vi "multiplexer.vi"() -> ()   [LabVIEW 2014]
uses:
  <vilib>/GPower/Numeric/GPNumeric.lvlib
panel:
  in  "LogFile":path
  in  "Logging Enabled?":bool
  # "\"mplexer data in\" - queue to receive data from sensors\n\"mplexer msg in\" - queue to send messages to multiplexer\n\"mplexer clock\" - notifier that will sound off every 25 ms, with an incrementing counter as a value; use it if you like.  Also, it will be canceled 10 ms after it sounds.\n\n\n\"mplexer msg out\" - none of your business!  (holds our subscribers - internal queue)"
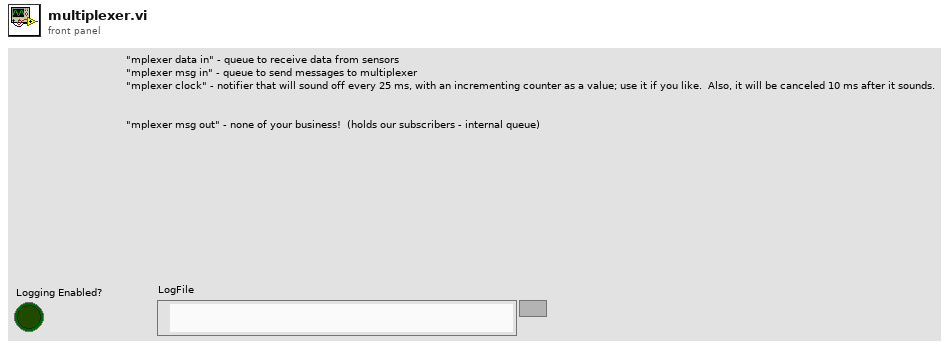
[diagram p1: front panel]
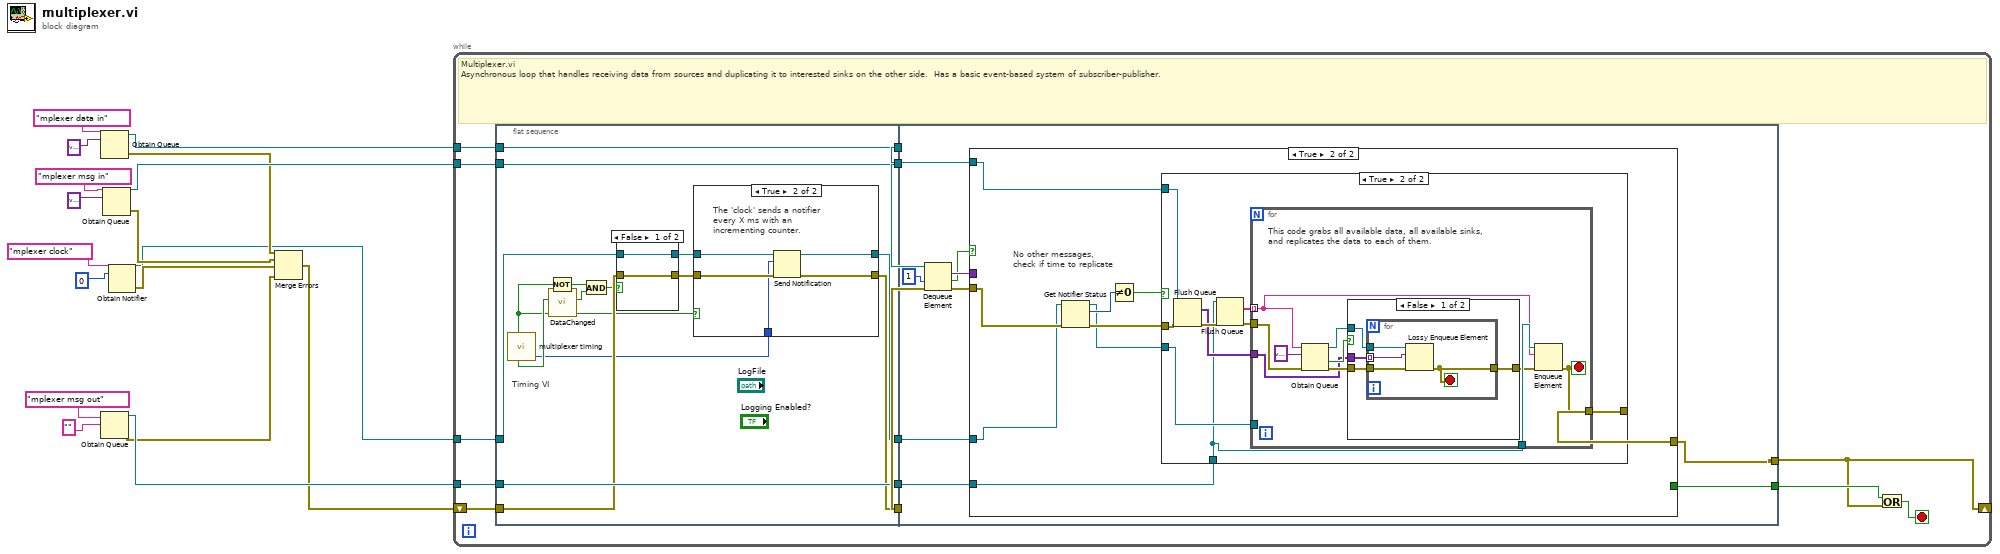
[diagram p0: block diagram]
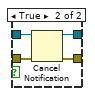
[diagram p2: hidden frame]
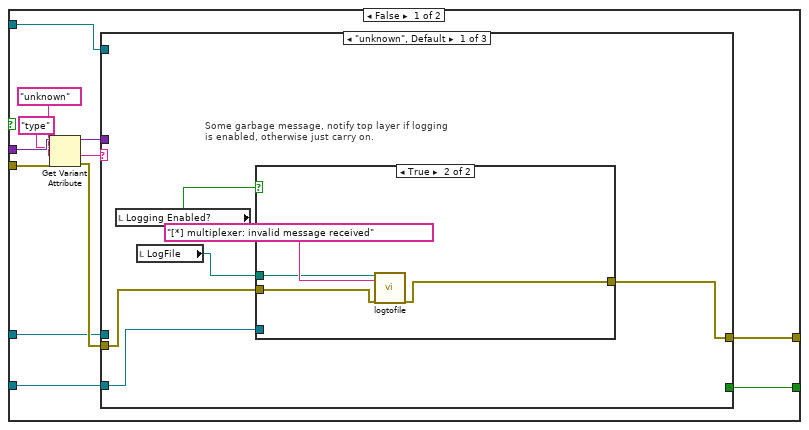
[diagram p4: hidden frame]
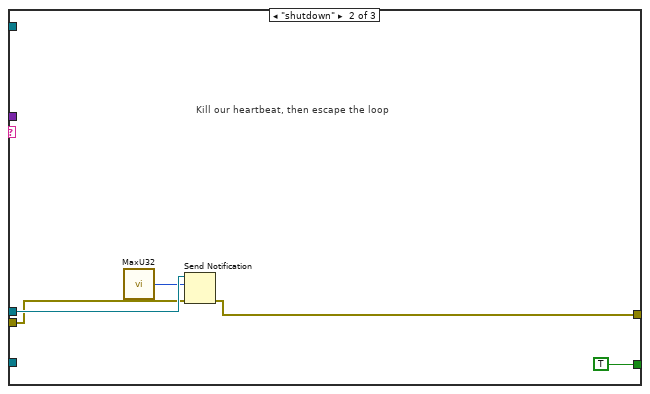
[diagram p6: hidden frame]
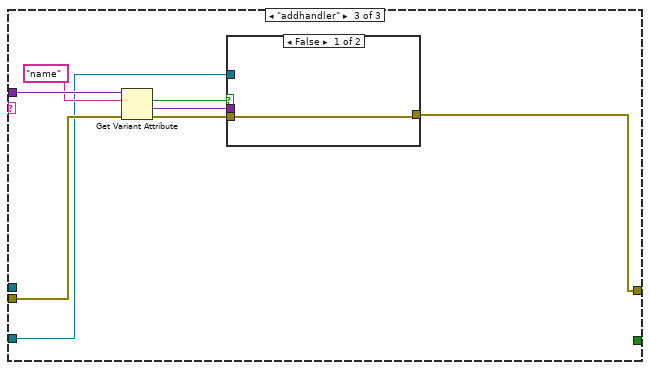
[diagram p7: hidden frame]
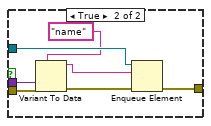
[diagram p8: hidden frame]
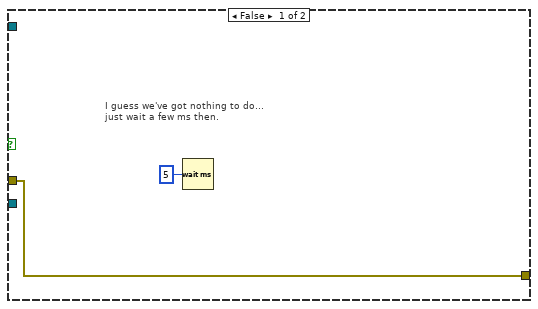
[diagram p9: hidden frame]
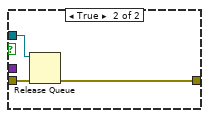
[diagram p10: hidden frame]
diagram:
  n1 = Obtain Queue(name (unnamed)="mplexer data in", element data type=variant) -> (queue out=w16:refnum<queue>, error out=w7:errorcluster)  [unwired: 3 in, 1 out]
  n2 = Obtain Queue(name (unnamed)="mplexer msg out", element data type="") -> (queue out=w13:refnum<queue>, error out=w1:errorcluster)  [unwired: 3 in, 1 out]
  n3 = Obtain Queue(name (unnamed)="mplexer msg in", element data type=variant) -> (queue out=w14:refnum<queue>, error out=w6:errorcluster)  [unwired: 3 in, 1 out]
  n4 = Obtain Notifier(name (unnamed)="mplexer clock", notification data type=u32 0) -> (notifier out=w3:refnum<notifier>, error out=w5:errorcluster)  [unwired: 2 in, 1 out]
  n5 = Merge Errors(w7, w6, w5, w1) -> (w4:errorcluster)
  n6 = while {
    tunnel: w16 -> [w20]
    shift-right: [w18] -> _
    shift-left: w4 -> [w28]
    tunnel: w14 -> [w25]
    tunnel: w13 -> [w26]
    tunnel: w3 -> [w23]
    stop <- w30 stop-if-true
    # "Multiplexer.vi\nAsynchronous loop that handles receiving data from sources and duplicating it to interested sinks on the other side.  Has a basic event-based system of subscriber-publisher."
    n7 = flat-sequence {
      tunnel: w28 -> [w40]
      tunnel: [w43] -> w29
      tunnel: [w44] -> w27
      tunnel: w26 -> [w44]
      tunnel: w25 -> [w45]
      tunnel: [w45] -> w24
      tunnel: w23 -> [w41]
      tunnel: [w32] -> w22
      tunnel: [w42] -> w21
      tunnel: w20 -> [w42]
      tunnel: w29 -> [w68]
      tunnel: w27 -> [w66]
      tunnel: w24 -> [w64]
      tunnel: [w62] -> w18
      tunnel: w22 -> [w61]
      tunnel: w21 -> [w60]
      tunnel: [w59] -> w19
      frame #0 {
        # "Timing VI"
        n8 = call "multiplexer timing.vi"() -> ("Clock Tick"=w36:bool, "Latch"=w37:bool, "Clock Counter"=w31:u32)  [unwired: 4 in, 2 out]
        n9 = Not(x=w36) -> (.not. x?=w35:bool)
        n10 = call <vilib>:"DataChanged.vi"("Data"=w37) -> ("Data changed?"=w34:bool)  [unwired: 10 in]
        n11 = And(x=w35, y=w34) -> (x .and. y?=w33:bool)
        n12 = case shown="False" w33 {
          tunnel: w41 -> [w46 w51]
          tunnel: w40 -> [w47 w50]
          tunnel: [w47 w49] -> w38
          tunnel: [w46 w48] -> w39
          frame False {
          }
          frame True {
            n13 = Cancel Notification(0:w51, 3:w50) -> (8:w48:refnum<notifier>, 11:w49:errorcluster)  [unwired: 1 out]
          }
        }
        n14 = case shown="True" w36 {
          tunnel: w39 -> [w53 w58]
          tunnel: [w52 w57] -> w43
          tunnel: w38 -> [w52 w56]
          tunnel: [w53 w55] -> w32
          tunnel: w31 -> [_ w54]
          frame False {
          }
          frame True {
            # "The 'clock' sends a notifier\nevery X ms with an\nincrementing counter."
            n15 = Send Notification(notification=w54, notifier=w58, error in (no error)=w56) -> (notifier out=w55:refnum<notifier>, error out=w57:errorcluster)
          }
        }
      }
      frame #1 {
        n16 = Dequeue Element(queue=w64, timeout in ms (-1)=1) -> (element=w65:variant, timed out?=w63:bool)  [unwired: 1 in, 2 out]
        n17 = case shown="True" w63 {
          tunnel: w68 -> [w78 w117]
          tunnel: w65 -> [w80 _]
          tunnel: w66 -> [w74 w113]
          tunnel: [w73 w112] -> w62
          tunnel: w61 -> [w71 w116]
          tunnel: w60 -> [w70 w115]
          tunnel: [w69 _] -> w59
          frame False {
            n18 = Get Variant Attribute(Variant=w80, name="type", default value (empty Variant)="unknown", error in=w78) -> (duplicate Variant=w72:variant, value=w75:string, error out=w76:errorcluster)  [unwired: 1 out]
            n19 = case shown="\"unknown\", Default" w75 {
              tunnel: w76 -> [w84 w94 w101]
              tunnel: w74 -> [w85 _ w99]
              tunnel: [w83 w92 w96] -> w73
              tunnel: w72 -> [_ _ w103]
              tunnel: w71 -> [_ w95 _]
              tunnel: w70 -> [_ _ _]
              tunnel: [_ TRUE _] -> w69
              frame "unknown", Default {
                # "Some garbage message, notify top layer if logging \nis enabled, otherwise just carry on."
                n20 = local read "Logging Enabled?"() -> (w82:bool)
                n21 = local read "LogFile"() -> (w81:path)
                n22 = case shown="True" w82 {
                  tunnel: w85 -> [_ _]
                  tunnel: w84 -> [w86 w88]
                  tunnel: [w86 w87] -> w83
                  tunnel: w81 -> [_ w89]
                  frame False {
                  }
                  frame True {
                    n23 = call "logtofile.vi"("LogFile"=w89, "text"="[*] multiplexer: invalid message received", "error in (no error)"=w88) -> ("error out"=w87:errorcluster)  [unwired: 16 in]
                  }
                }
              }
              frame "shutdown" {
                # "Kill our heartbeat, then escape the loop"
                n24 = call <vilib>:"MaxU32.vi"() -> ("Maximum value"=w93:u32)
                n25 = Send Notification(notification=w93, notifier=w95, error in (no error)=w94) -> (error out=w92:errorcluster)  [unwired: 1 out]
              }
              frame "addhandler" {
                n26 = Get Variant Attribute(Variant=w103, name="name", error in=w101) -> (found=w100:bool, value=w98:variant, error out=w97:errorcluster)  [unwired: 1 in, 1 out]
                n27 = case shown="False" w100 {
                  tunnel: w99 -> [_ w111]
                  tunnel: w98 -> [_ w110]
                  tunnel: w97 -> [w104 w106]
                  tunnel: [w104 w107] -> w96
                  frame False {
                  }
                  frame True {
                    n28 = Variant To Data(error in=w106, type="name" ("name"), Variant=w110) -> (data=w108:string, error out=w105:errorcluster)
                    n29 = Enqueue Element(queue=w111, element=w108, error in (no error)=w105) -> (error out=w107:errorcluster)  [unwired: 1 in, 2 out]
                  }
                }
              }
            }
          }
          frame True {
            # "No other messages,\ncheck if time to replicate"
            n30 = Get Notifier Status(notifier=w116, error in (no error)=w117) -> (notifier out=w114:refnum<notifier>, current notification=w120:u32, error out=w118:errorcluster)  [unwired: 2 out]
            n31 = Not Equal To 0?(x=w120) -> (x != 0?=w119:bool)
            n32 = case shown="True" w119 {
              tunnel: w118 -> [w122 w128]
              tunnel: w115 -> [_ w129]
              tunnel: [w122 w125] -> w112
              tunnel: w114 -> [_ w124]
              tunnel: w113 -> [_ w123]
              frame False {
                # "I guess we've got nothing to do...\njust wait a few ms then."
                n33 = Wait (ms)(milliseconds to wait=u32 5) -> ()  [unwired: 1 out]
              }
              frame True {
                n34 = Flush Queue(queue=w129, error in (no error)=w128) -> (remaining elements=w126:variant[], error out=w127:errorcluster)  [unwired: 1 out]
                n35 = Flush Queue(queue=w123, error in (no error)=w127) -> (remaining elements=w130:string[], error out=w131:errorcluster)  [unwired: 1 out]
                n36 = for {
                  tunnel: w131 -> [w141]
                  tunnel: w130 -> [w134] mode=indexing
                  tunnel: w124 -> [_]
                  tunnel: w126 -> [w136]
                  tunnel: [w132] -> w125
                  tunnel: w123 -> [w135]
                  stop <- w132 stop-if-true
                  # "This code grabs all available data, all available sinks,\nand replicates the data to each of them."
                  n37 = Obtain Queue(name (unnamed)=w134, element data type=variant, error in (no error)=w141) -> (queue out=w137:refnum<queue>, created new?=w139:bool, error out=w138:errorcluster)  [unwired: 2 in]
                  n38 = case shown="False" w139 {
                    tunnel: w138 -> [w143 w151]
                    tunnel: w137 -> [w144 w152]
                    tunnel: [w142 w150] -> w133
                    tunnel: w136 -> [w145 _]
                    frame False {
                      n39 = for {
                        tunnel: w145 -> [w149] mode=indexing
                        tunnel: w144 -> [w148]
                        tunnel: w143 -> [w147]
                        tunnel: [w146] -> w142
                        stop <- w146 stop-if-true
                        n40 = Lossy Enqueue Element(queue=w148, element=w149, error in (no error)=w147) -> (error out=w146:errorcluster)  [unwired: 3 out]
                      }
                    }
                    frame True {
                      n41 = Release Queue(queue=w152, error in (no error)=w151) -> (error out=w150:errorcluster)  [unwired: 1 in, 2 out]
                    }
                  }
                  n42 = Enqueue Element(queue=w135, element=w134, error in (no error)=w133) -> (error out=w132:errorcluster)  [unwired: 1 in, 2 out]
                }
              }
            }
          }
        }
      }
    }
    n43 = Or(x=w19, y=w18) -> (x .or. y?=w30:bool)
  }
